vi "Add Task.vi"(8 "error in (no error)":errorcluster, 10 "Analog Configuration Parameters":T1, 11 "Analog Input in":refnum<class "Analog Input.lvclass">) -> (0 "error out":errorcluster, 3 "Analog Input out":refnum<class "Analog Input.lvclass">)   [LabVIEW 2021, in "Analog Input.lvlib" / "Analog Input.lvclass"]
uses:
  Analog Input.lvclass
  Analog Input.lvclass/Analog Input.ctl
  <vilib>/DAQmx/create/channels.llb/DAQmx Create Channel (AI-Voltage-Basic).vi
  Utilities/Analog Configuration Parameters.ctl
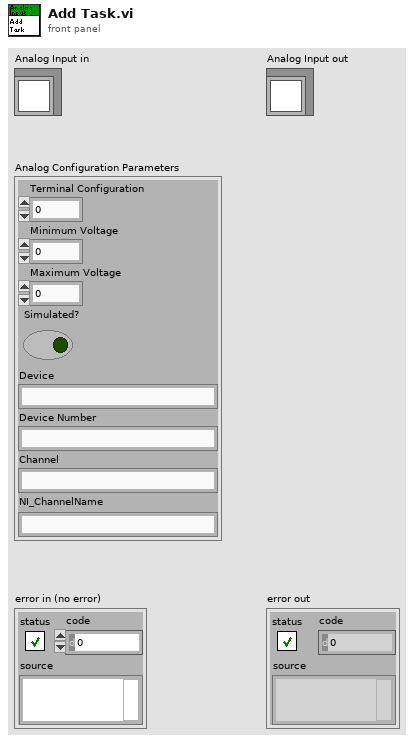
[diagram p1: front panel]
types:
  T1 = typedef "Analog Configuration Parameters.ctl" = cluster{"Terminal Configuration":i32, "Minimum Voltage":dbl, "Maximum Voltage":dbl, "Simulated?":bool, "Device":string, "Device Number":string, "Channel":string, "NI_ChannelName":string}
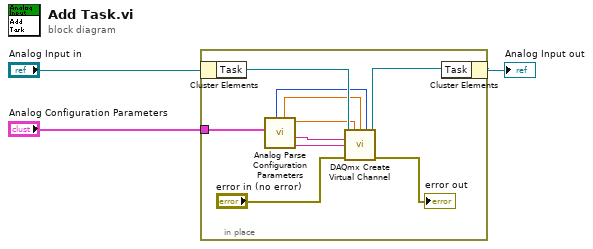
[diagram p0: block diagram]
diagram:
  n1 = in-place {
    in-place-border: "Analog Configuration Parameters" -> [w4]
    n2 = in-place-cluster #1("Analog Input in") -> ("Task"=w13:refnum<k21>)
    n3 = call "Analog Parse Configuration Parameters.vi"("Analog Configuration Parameters"=w4) -> ("name to assign"=w11:string, "physical channels"=w10:string, "Maximum Voltage"=w9:dbl, "Minimum Voltage"=w8:dbl, "Terminal Configuration"=w7:i32)  [unwired: 6 in]
    n4 = call-poly <vilib>:"DAQmx Create Virtual Channel.vi"("task in"=w13, "maximum value"=w9, "minimum value"=w8, "input terminal configuration"=w7, "physical channels"=w10, "name to assign"=w11, "error in"="error in (no error)") -> ("task out"=w12:refnum<k21>, "error out"=→"error out":errorcluster)  [unwired: 7 in]
    n5 = in-place-cluster #1("Task"=w12) -> (→"Analog Input out":refnum<class "Analog Input.lvclass">)
  }
